vi "Project 5 - Johnson.vi"() -> ()   [LabVIEW 2019]
uses:
  <vilib>/Utility/file.llb/Read Delimited Spreadsheet (string).vi
  <vilib>/Utility/file.llb/Write Delimited Spreadsheet (string).vi
panel:
  out "user match?":bool
  out "Row found":i32
  out "x = y?":bool[](array[boolean])
  out "Tab Control":enum32{"Login", "S.H.I.T", "Database"}(tab)
  in  "ENTER Button":bool
  in  "Name":string
  in  "ID":string
  in  "Pin":string
  in  "stop":bool
  out "User Logged In":string
  in  "LOGOUT Button":bool
  in  "Database Button":bool
  in  "Simulate Button":bool
  out "Collected Signals":dynamicdata(graph)
  in  "Save Button":bool
  in  "all rows":string[][](array[string])=[["Name", "OU ID", "PIN", "Type"], ["Bud Wilkinson", "111-11-1111", "1956", "user"], ["Barry Switzer", "118-45-1975", "1985", "user"], ["Bob Stoops", "113-45-6789", "2000", "user"], ["Lincoln Riley", "777-77-7777", "2020", "user"], ["Chad Davis", "123-45-6789", "1234", "admin"], ["Matt Johnson", "000-00-0000", "0000", "admin"], ["Matt Johnson", "000-00-0000", "0001", "aDMiN"], ["Matt Johnson", "000-00-0000", "0002", "ADMIN"], ["Matt Johnson", "000-00-0000", "0003", "AdmiN"]]
  in  "S.H.I.T. Button":bool
  in  "Open File Button":bool
  # "S.H.I.T. Login"
  # "S.H.I.T.base"
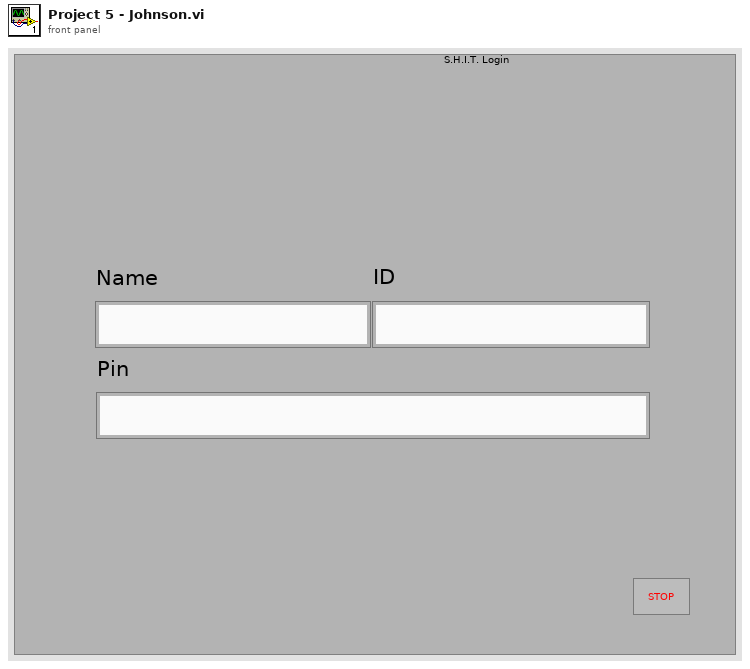
[diagram p1: front panel]
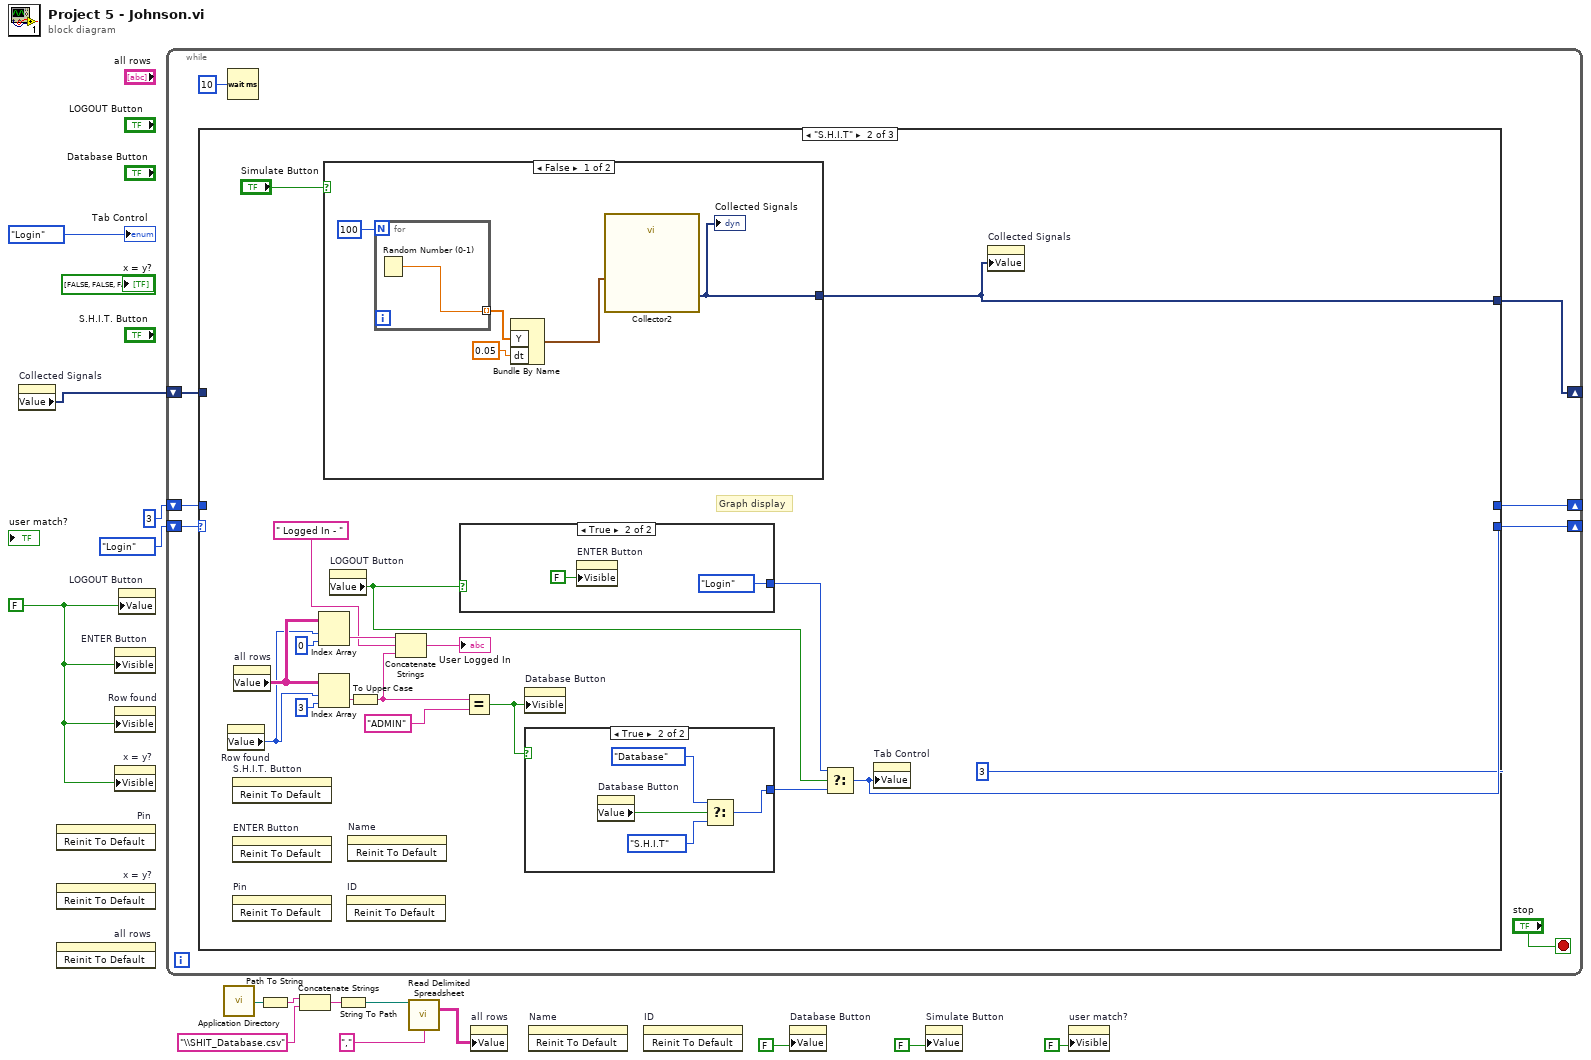
[diagram p0: block diagram]
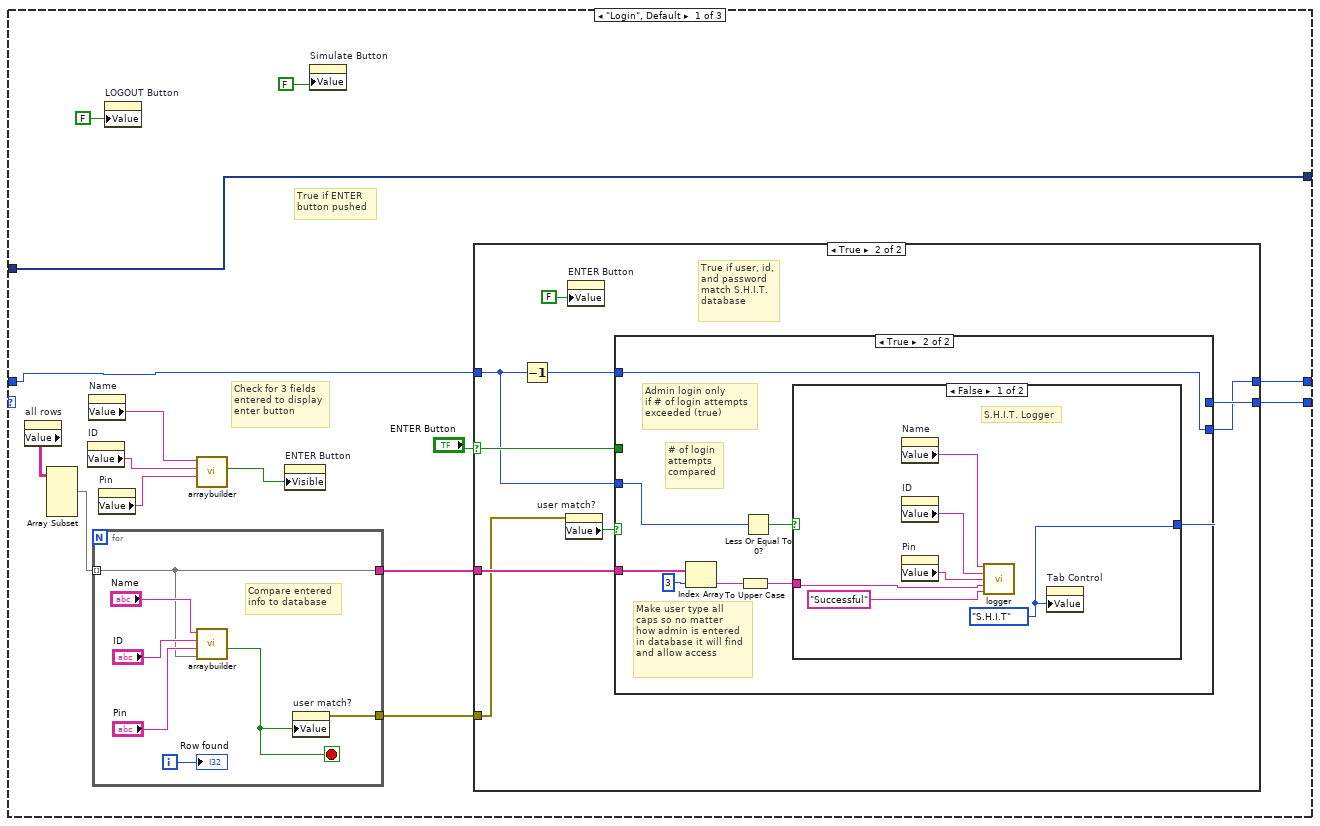
[diagram p2: hidden frame]
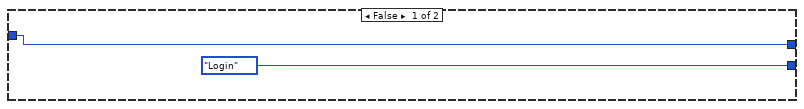
[diagram p3: hidden frame]
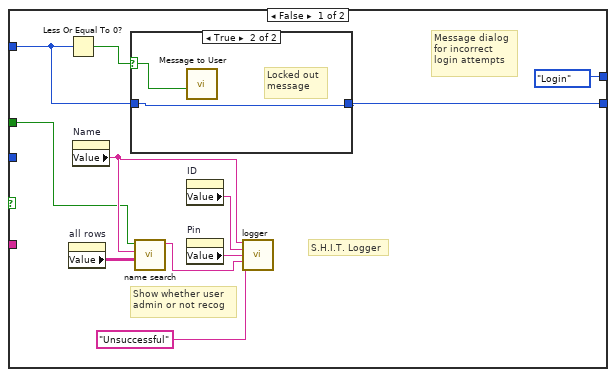
[diagram p4: hidden frame]
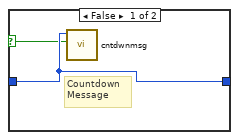
[diagram p5: hidden frame]
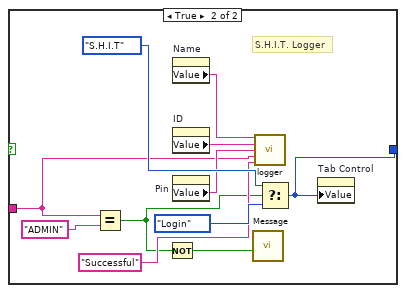
[diagram p6: hidden frame]
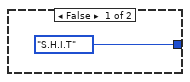
[diagram p7: hidden frame]
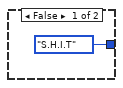
[diagram p8: hidden frame]
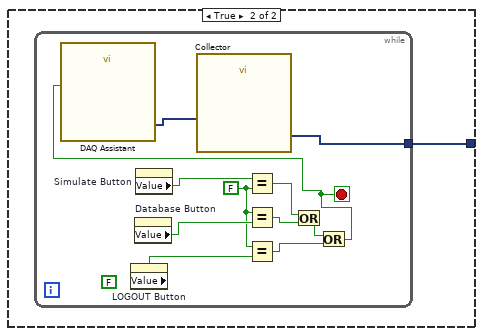
[diagram p9: hidden frame]
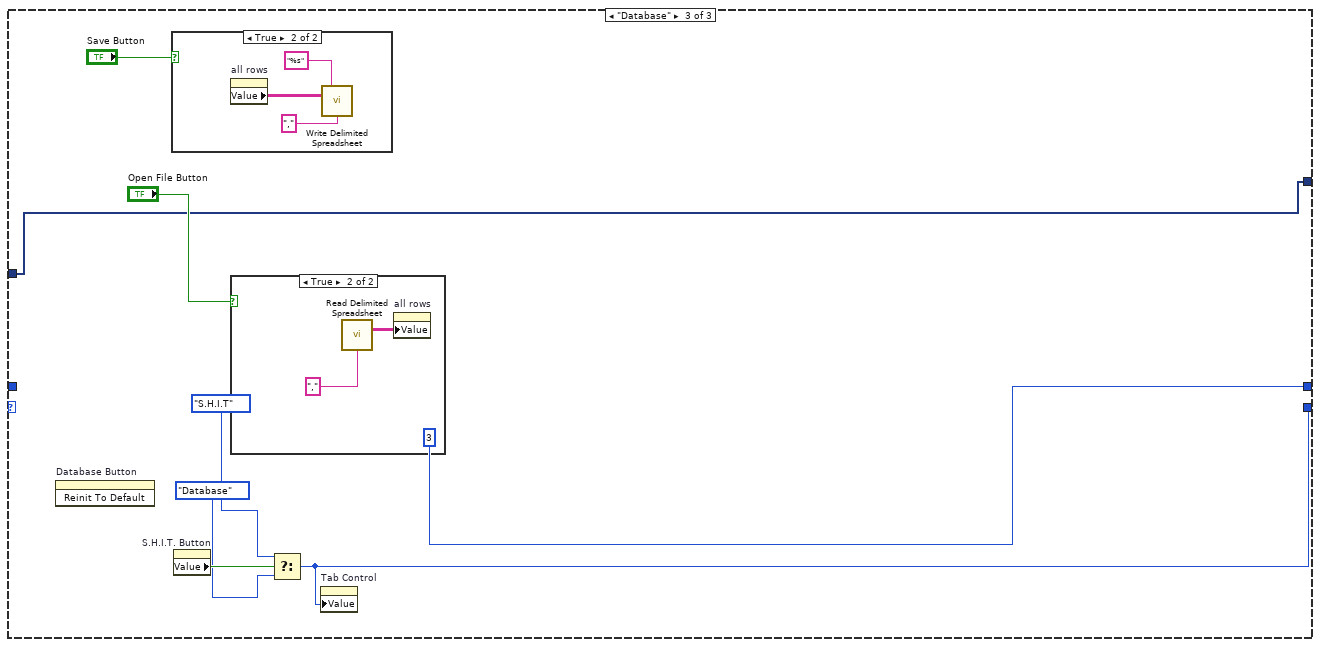
[diagram p10: hidden frame]
diagram:
  w3 = FALSE ("LOGOUT Button")
  n1 = property on="Collected Signals" class="WFGraph (strict)"() -> ("Value"=w1:dynamicdata)  [unwired: 2 in, 2 out]
  n2 = invoke on="Pin" class="Str" method="Reinit To Default"() -> ()  [unwired: 3 in, 3 out]
  n3 = invoke on="x = y?" class="Arr (strict)" method="Reinit To Default"() -> ()  [unwired: 3 in, 3 out]
  n4 = invoke on="all rows" class="Arr (strict)" method="Reinit To Default"() -> ()  [unwired: 3 in, 3 out]
  n5 = property on="ENTER Button" class="Bool (strict)"("Visible"=w3) -> ()  [unwired: 2 in, 2 out]
  n6 = property on="Row found" class="DigNum (strict)"("Visible"=w3) -> ()  [unwired: 2 in, 2 out]
  n7 = property on="x = y?" class="Arr (strict)"("Visible"=w3) -> ()  [unwired: 2 in, 2 out]
  n8 = property on="LOGOUT Button" class="Bool (strict)"("Value"=w3) -> ()  [unwired: 2 in, 2 out]
  n9 = while {
    shift-right: [w21] -> _
    shift-left: enum32{"Login", "S.H.I.T", "Database"}."Login" ("Tab Control") -> [w22]
    shift-right: [w19] -> _
    shift-left: 3 -> [w20]
    shift-right: [w18] -> _
    shift-left: w1 -> [w17]
    stop <- "stop" stop-if-true
    n10 = case shown="\"S.H.I.T\"" w22 {
      tunnel: [w38 w110 w146] -> w21
      tunnel: w20 -> [w36 _ _]
      tunnel: [w35 3 3] -> w19
      tunnel: [w25 w98 w142] -> w18
      tunnel: w17 -> [w25 _ w142]
      frame "Login", Default {
        # "True if ENTER\nbutton pushed"
        # "Check for 3 fields\nentered to display\nenter button"
        n11 = property on="all rows" class="Arr (strict)"() -> ("Value"=w39:string[][])  [unwired: 2 in, 2 out]
        n12 = Array Subset(array=w39) -> (w32:string[][])  [unwired: 4 in]
        n13 = property on="ID" class="Str"() -> ("Value"=w28:string)  [unwired: 2 in, 2 out]
        n14 = property on="Name" class="Str"() -> ("Value"=w27:string)  [unwired: 2 in, 2 out]
        n15 = for {
          tunnel: w32 -> [w92] mode=indexing
          tunnel: [w92] -> w34
          tunnel: [w97] -> w30
          i -> [w96]
          stop <- w91 stop-if-true
          # "Compare entered\ninfo to database"
          n16 = call "arraybuilder.vi"("Array"=w92, "Pin"="Pin", "ID"="ID", "Name"="Name") -> ("User match"=w91:bool)  [unwired: 6 in, 1 out]
          n17 = property on="user match?" class="Bool (strict)"("Value"=w91) -> (error out=w97:errorcluster)  [unwired: 2 in, 1 out]
          "Row found" <- w96
        }
        n18 = property on="Pin" class="Str"() -> ("Value"=w29:string)  [unwired: 2 in, 2 out]
        n19 = property on="LOGOUT Button" class="Bool (strict)"("Value"=FALSE ("LOGOUT Button")) -> ()  [unwired: 2 in, 2 out]
        n20 = call "arraybuilder.vi"("Pin"=w29, "ID"=w28, "Name"=w27) -> ("Fields entered"=w31:bool)  [unwired: 7 in, 1 out]
        n21 = property on="ENTER Button" class="Bool (strict)"("Visible"=w31) -> ()  [unwired: 2 in, 2 out]
        n22 = property on="Simulate Button" class="Bool (strict)"("Value"=FALSE ("Simulate Button")) -> ()  [unwired: 2 in, 2 out]
        n23 = case shown="True" "ENTER Button" {
          selector: "ENTER Button" -> [_ w45]
          tunnel: [enum32{"Login", "S.H.I.T", "Database"}."Login" ("Tab Control") w50] -> w38
          tunnel: w36 -> [w40 w44]
          tunnel: [w40 w49] -> w35
          tunnel: w34 -> [_ w48]
          tunnel: w30 -> [_ w42]
          frame False {
          }
          frame True {
            # "True if user, id,\nand password\nmatch S.H.I.T.\ndatabase"
            n24 = Decrement(x=w44) -> (x-1=w47:i32)
            n25 = property on="user match?" class="Bool (strict)"(error in=w42) -> ("Value"=w43:bool)  [unwired: 1 in, 2 out]
            n26 = property on="ENTER Button" class="Bool (strict)"("Value"=FALSE ("ENTER Button")) -> ()  [unwired: 2 in, 2 out]
            n27 = case shown="True" w43 {
              tunnel: [enum32{"Login", "S.H.I.T", "Database"}."Login" ("Tab Control") w69] -> w50
              tunnel: w47 -> [w58 w66]
              tunnel: [w59 w66] -> w49
              tunnel: w48 -> [_ w72]
              tunnel: w45 -> [w51 _]
              tunnel: w44 -> [_ w68]
              frame False {
                # "Message dialog\nfor incorrect\nlogin attempts"
                # "S.H.I.T. Logger"
                # "Show whether user\nadmin or not recog"
                n28 = Less Or Equal To 0?(x=w58) -> (x <= 0?=w60:bool)
                n29 = property on="all rows" class="Arr (strict)"() -> ("Value"=w56:string[][])  [unwired: 2 in, 2 out]
                n30 = property on="Name" class="Str"() -> ("Value"=w54:string)  [unwired: 2 in, 2 out]
                n31 = case shown="True" w60 {
                  selector: w60 -> [w62 w65]
                  tunnel: w58 -> [w63 w64]
                  tunnel: [w63 w64] -> w59
                  frame False {
                    # "Countdown\nMessage"
                    n32 = call "cntdwnmsg.vi"("Boolean"=w62, "Numeric"=w63) -> ()  [unwired: 10 in]
                  }
                  frame True {
                    # "Locked out\nmessage"
                    n33 = call "Message to User"("Enable"=w65) -> ()  [unwired: 9 in, 2 out]
                  }
                }
                n34 = call "name search.vi"("Value 2"=w56, "Value"=w54, "Value 3"=w51) -> ("User/Admin"=w55:string)  [unwired: 8 in]
                n35 = property on="ID" class="Str"() -> ("Value"=w53:string)  [unwired: 2 in, 2 out]
                n36 = property on="Pin" class="Str"() -> ("Value"=w52:string)  [unwired: 2 in, 2 out]
                n37 = call "logger.vi"("Name"=w54, "ID"=w53, "Pin"=w52, "User/Admin"=w55, "Success?"="Unsuccessful") -> ()  [unwired: 11 in]
              }
              frame True {
                # "# of login\nattempts\ncompared"
                # "Make user type all\ncaps so no matter\nhow admin is entered\nin database it will find\nand allow access"
                # "Admin login only\nif # of login attempts\nexceeded (true)"
                n38 = Index Array(array=w72, index=3) -> (element=w70:string)
                n39 = To Upper Case(1:w70) -> (0:w67:string)
                n40 = Less Or Equal To 0?(x=w68) -> (x <= 0?=w73:bool)
                n41 = case shown="False" w73 {
                  tunnel: [w79 w88] -> w69
                  tunnel: w67 -> [w77 w81]
                  frame False {
                    w79 = enum32{"Login", "S.H.I.T", "Database"}."S.H.I.T" ("Tab Control")
                    # "S.H.I.T. Logger"
                    n42 = property on="Name" class="Str"() -> ("Value"=w76:string)  [unwired: 2 in, 2 out]
                    n43 = property on="ID" class="Str"() -> ("Value"=w75:string)  [unwired: 2 in, 2 out]
                    n44 = property on="Pin" class="Str"() -> ("Value"=w74:string)  [unwired: 2 in, 2 out]
                    n45 = call "logger.vi"("Name"=w76, "ID"=w75, "Pin"=w74, "User/Admin"=w77, "Success?"="Successful") -> ()  [unwired: 11 in]
                    n46 = property on="Tab Control" class="TabCtl (strict)"("Value"=w79) -> ()  [unwired: 2 in, 2 out]
                  }
                  frame True {
                    # "S.H.I.T. Logger"
                    n47 = Equal?(x=w81, y="ADMIN") -> (x = y?=w80:bool)
                    n48 = Not(x=w80) -> (.not. x?=w87:bool)
                    n49 = property on="Name" class="Str"() -> ("Value"=w85:string)  [unwired: 2 in, 2 out]
                    n50 = property on="ID" class="Str"() -> ("Value"=w84:string)  [unwired: 2 in, 2 out]
                    n51 = property on="Pin" class="Str"() -> ("Value"=w83:string)  [unwired: 2 in, 2 out]
                    n52 = call "Message"("Enable"=w87) -> ()  [unwired: 9 in, 2 out]
                    n53 = call "logger.vi"("Name"=w85, "ID"=w84, "Pin"=w83, "User/Admin"=w81, "Success?"="Successful") -> ()  [unwired: 11 in]
                    n54 = Select(t=enum32{"Login", "S.H.I.T", "Database"}."S.H.I.T" ("Tab Control"), s=w80, f=enum32{"Login", "S.H.I.T", "Database"}."Login" ("Tab Control")) -> (s? t:f=w88:enum32{"Login", "S.H.I.T", "Database"})
                    n55 = property on="Tab Control" class="TabCtl (strict)"("Value"=w88) -> ()  [unwired: 2 in, 2 out]
                  }
                }
              }
            }
          }
        }
      }
      frame "S.H.I.T" {
        # "Graph display"
        n56 = property on="Row found" class="DigNum (strict)"() -> ("Value"=w108:i32)  [unwired: 2 in, 2 out]
        n57 = invoke on="S.H.I.T. Button" class="Bool (strict)" method="Reinit To Default"() -> ()  [unwired: 3 in, 3 out]
        n58 = invoke on="ENTER Button" class="Bool (strict)" method="Reinit To Default"() -> ()  [unwired: 3 in, 3 out]
        n59 = invoke on="Pin" class="Str" method="Reinit To Default"() -> ()  [unwired: 3 in, 3 out]
        n60 = property on="all rows" class="Arr (strict)"() -> ("Value"=w109:string[][])  [unwired: 2 in, 2 out]
        n61 = Index Array(array=w109, index (row)=w108, index (col)=0 ("disabled index (col)")) -> (element=w106:string)
        n62 = Index Array(array=w109, index (row)=w108, index (col)=3 ("disabled index (col)")) -> (element=w104:string)
        n63 = case shown="False" "Simulate Button" {
          tunnel: [w124 w130] -> w98
          frame False {
            n64 = for {
              N: 100 -> [_]
              tunnel: [w129] -> w126 mode=indexing
              n65 = Random Number (0-1)() -> (number: 0 to 1=w129:dbl)
            }
            n66 = Bundle By Name("Y"=w126, "dt"=0.05) -> (w125:waveform(dbl))  [unwired: 1 in]
            n67 = call "Collector2"("Signals"=w125) -> ("Collected Signals"=w124:dynamicdata)  [unwired: 9 in, 1 out]
            "Collected Signals" <- w124
          }
          frame True {
            n68 = while {
              tunnel: [w131] -> w130
              stop <- w132 stop-if-true
              (unwired) FALSE ("Database Button")
              w138 = FALSE ("y")
              n69 = property on="LOGOUT Button" class="Bool (strict)"() -> ("Value"=w137:bool)  [unwired: 2 in, 2 out]
              n70 = property on="Database Button" class="Bool (strict)"() -> ("Value"=w139:bool)  [unwired: 2 in, 2 out]
              n71 = property on="Simulate Button" class="Bool (strict)"() -> ("Value"=w141:bool)  [unwired: 2 in, 2 out]
              n72 = Equal?(x=w141, y=w138) -> (x = y?=w140:bool)
              n73 = Equal?(x=w138, y=w139) -> (x = y?=w136:bool)
              n74 = Equal?(x=w138, y=w137) -> (x = y?=w134:bool)
              n75 = Or(x=w140, y=w136) -> (x .or. y?=w135:bool)
              n76 = Or(x=w135, y=w134) -> (x .or. y?=w132:bool)
              n77 = call "DAQ Assistant"("stop (F)"=w132) -> ("data"=w133:dynamicdata)  [unwired: 15 in, 3 out]
              n78 = call "Collector"("Signals"=w133) -> ("Collected Signals"=w131:dynamicdata)  [unwired: 9 in, 1 out]
            }
          }
        }
        n79 = property on="LOGOUT Button" class="Bool (strict)"() -> ("Value"=w100:bool)  [unwired: 2 in, 2 out]
        n80 = invoke on="ID" class="Str" method="Reinit To Default"() -> ()  [unwired: 3 in, 3 out]
        n81 = invoke on="Name" class="Str" method="Reinit To Default"() -> ()  [unwired: 3 in, 3 out]
        n82 = To Upper Case(1:w104) -> (0:w99:string)
        n83 = Concatenate Strings(w106, " Logged In - " ("string"), w99) -> (→"User Logged In":string)
        n84 = case shown="True" w100 {
          tunnel: [enum32{"Login", "S.H.I.T", "Database"}."S.H.I.T" ("Tab Control") enum32{"Login", "S.H.I.T", "Database"}."Login" ("Tab Control")] -> w111
          frame False {
          }
          frame True {
            n85 = property on="ENTER Button" class="Bool (strict)"("Visible"=FALSE) -> ()  [unwired: 2 in, 2 out]
          }
        }
        n86 = Equal?(x=w99, y="ADMIN") -> (x = y?=w113:bool)
        n87 = property on="Database Button" class="Bool (strict)"("Visible"=w113) -> ()  [unwired: 2 in, 2 out]
        n88 = case shown="True" w113 {
          tunnel: [enum32{"Login", "S.H.I.T", "Database"}."S.H.I.T" ("Tab Control") w120] -> w112
          frame False {
          }
          frame True {
            n89 = property on="Database Button" class="Bool (strict)"() -> ("Value"=w123:bool)  [unwired: 2 in, 2 out]
            n90 = Select(t=enum32{"Login", "S.H.I.T", "Database"}."Database" ("Tab Control"), s=w123, f=enum32{"Login", "S.H.I.T", "Database"}."S.H.I.T" ("Tab Control")) -> (s? t:f=w120:enum32{"Login", "S.H.I.T", "Database"})
          }
        }
        n91 = Select(t=w111, s=w100, f=w112) -> (s? t:f=w110:enum32{"Login", "S.H.I.T", "Database"})
        n92 = property on="Tab Control" class="TabCtl (strict)"("Value"=w110) -> ()  [unwired: 2 in, 2 out]
        n93 = property on="Collected Signals" class="WFGraph (strict)"("Value"=w98) -> ()  [unwired: 2 in, 2 out]
      }
      frame "Database" {
        n94 = invoke on="Database Button" class="Bool (strict)" method="Reinit To Default"() -> ()  [unwired: 3 in, 3 out]
        n95 = case shown="True" "Save Button" {
          frame False {
          }
          frame True {
            n96 = property on="all rows" class="Arr (strict)"() -> ("Value"=w152:string[][])  [unwired: 2 in, 2 out]
            n97 = call-poly <vilib>:"Write Delimited Spreadsheet.vi"("format (%s)"="%s" ("format (%.3f)"), "2D data"=w152, "delimiter (\\t)"="," ("delimiter (\\t)")) -> ()  [unwired: 11 in, 2 out]
          }
        }
        n98 = property on="S.H.I.T. Button" class="Bool (strict)"() -> ("Value"=w149:bool)  [unwired: 2 in, 2 out]
        n99 = case shown="True" "Open File Button" {
          frame False {
          }
          frame True {
            n100 = call-poly <vilib>:"Read Delimited Spreadsheet.vi"("delimiter (\\t)"="," ("delimiter (\\t)")) -> ("all rows"=w150:string[][])  [unwired: 9 in, 5 out]
            n101 = property on="all rows" class="Arr (strict)"("Value"=w150) -> ()  [unwired: 2 in, 2 out]
          }
        }
        n102 = Select(t=enum32{"Login", "S.H.I.T", "Database"}."S.H.I.T" ("Tab Control"), s=w149, f=enum32{"Login", "S.H.I.T", "Database"}."Database" ("Tab Control")) -> (s? t:f=w146:enum32{"Login", "S.H.I.T", "Database"})
        n103 = property on="Tab Control" class="TabCtl (strict)"("Value"=w146) -> ()  [unwired: 2 in, 2 out]
      }
    }
    n104 = Wait (ms)(milliseconds to wait=u32 10) -> ()  [unwired: 1 out]
  }
  n105 = call <vilib>:"Application Directory.vi"() -> ("Application Directory"=w16:path)
  n106 = Path To String(path=w16) -> (string=w15:string)
  n107 = Concatenate Strings(w15, "\\SHIT_Database.csv" ("string")) -> (w13:string)
  n108 = String To Path(string=w13) -> (path=w12:path)
  n109 = call-poly <vilib>:"Read Delimited Spreadsheet.vi"("file path (dialog if empty)"=w12, "delimiter (\\t)"="," ("delimiter (\\t)")) -> ("all rows"=w4:string[][])  [unwired: 8 in, 5 out]
  n110 = property on="all rows" class="Arr (strict)"("Value"=w4) -> ()  [unwired: 2 in, 2 out]
  n111 = invoke on="Name" class="Str" method="Reinit To Default"() -> ()  [unwired: 3 in, 3 out]
  n112 = invoke on="ID" class="Str" method="Reinit To Default"() -> ()  [unwired: 3 in, 3 out]
  n113 = property on="Database Button" class="Bool (strict)"("Value"=FALSE ("Database Button")) -> ()  [unwired: 2 in, 2 out]
  n114 = property on="Simulate Button" class="Bool (strict)"("Value"=FALSE ("Simulate Button")) -> ()  [unwired: 2 in, 2 out]
  n115 = property on="user match?" class="Bool (strict)"("Visible"=FALSE) -> ()  [unwired: 2 in, 2 out]
  "Tab Control" <- enum32{"Login", "S.H.I.T", "Database"}."Login" ("Tab Control")
  "x = y?" <- bool[] [FALSE, FALSE, FALSE] ("x = y? 2")
